vi "setAverage.vi"(8 "error in (no error)":errorcluster, 9 "Average Factor":i32, 10 "Average?":enum16{"ON", "OFF"}(ring), 11 "Instrument.VSource in":refnum<class "Instrument.VNA.lvclass">) -> (0 "error out":errorcluster, 3 "Instrument.VSource out":refnum<class "Instrument.VNA.lvclass">)   [LabVIEW 2019, in "Instrument.VNA.lvclass"]
uses:
  Instrument.VNA.lvclass
  C:/Users/patrick/Documents/GitHub/Instrument-Framework/lvsrc/Framework/Instrument/Instrument.lvclass
  Typedefs/setAverage--cluster.ctl
  Typedefs/VNA.Commands--Enum.ctl
  Instrument/Instrument.lvclass
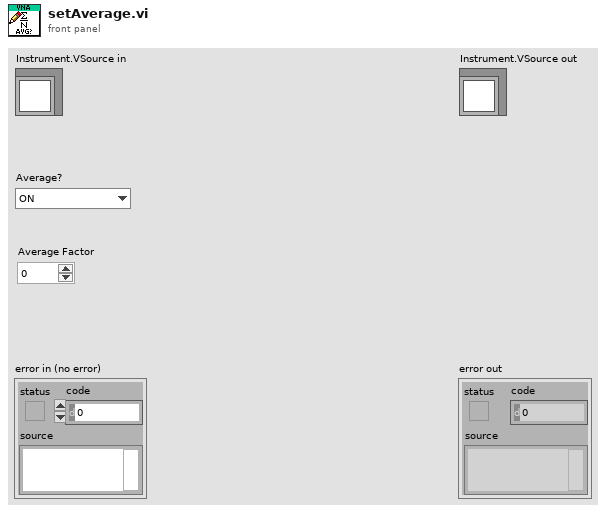
[diagram p1: front panel]
types:
  T1 = typedef "Instrument.VNA.lvclass/VNA.Commands--Enum.ctl" = enum16{"getData", "setAverage", "setFormat", "setMeasurement", "setPower", "setSweep"}
  T2 = typedef "Instrument.VNA.lvclass/setAverage--cluster.ctl" = cluster{"average":enum16{"ON", "OFF"}, "factor":i32}
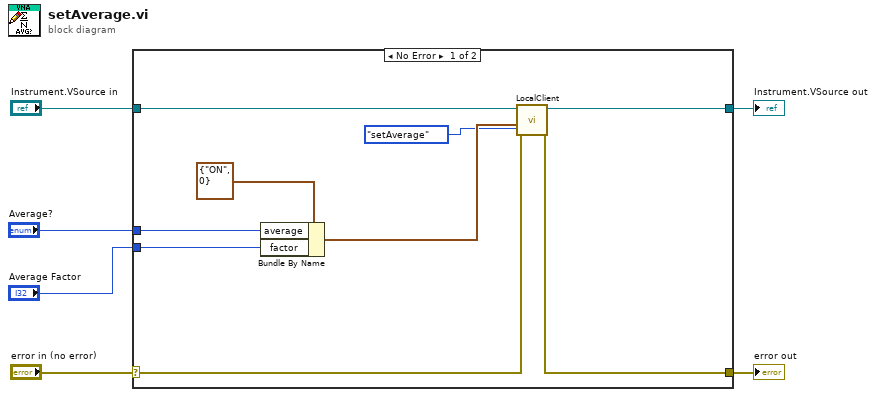
[diagram p0: block diagram]
diagram:
  n1 = case shown="No Error" "error in (no error)" {
    selector: "error in (no error)" -> [w8 w17]
    tunnel: [w14 w17] -> w5
    tunnel: [w15 w16] -> w3
    tunnel: "Instrument.VSource in" -> [w9 w16]
    tunnel: "Average Factor" -> [w12 _]
    tunnel: "Average?" -> [w11 _]
    frame No Error {
      n2 = Bundle By Name(cluster=T2 {"average"=enum."ON", "factor"=0} ("setAverage"), "average"=w11, "factor"=w12) -> (w10:T2)
      n3 = call "LocalClient.vi"("timeout (ms) [500]"=VNA.Commands--Enum."setAverage" ("Commands"), "error in (no error)"=w8, "params"=w10, "Instrument in"=w9) -> ("error out"=w14:errorcluster, "Instrument out"=w15:refnum<class "Instrument.VNA.lvclass">)  [unwired: 4 in, 2 out]
    }
    frame Error {
    }
  }
  "error out" <- w5
  "Instrument.VSource out" <- w3
